vi "Get Torque.vi"(8 "error in (no error)":errorcluster, 11 "HSU MCU V2 in":refnum<class "HSU MCU V2.lvclass">) -> (0 "error out":errorcluster, 2 "Torque":dbl, 3 "HSU MCU V2 out":refnum<class "HSU MCU V2.lvclass">)   [LabVIEW 2024, in "HSU MCU V2.lvclass"]
uses:
  HSU MCU V2.lvclass
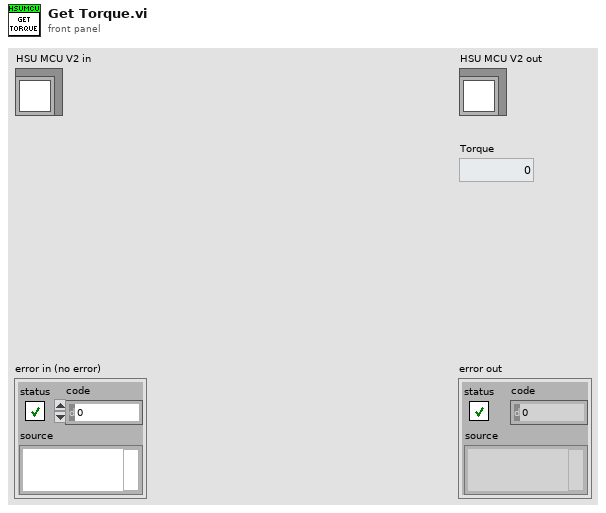
[diagram p1: front panel]
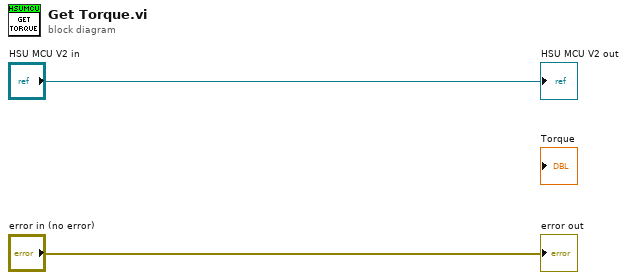
[diagram p0: block diagram]
diagram:
  "error out" <- "error in (no error)"
  "HSU MCU V2 out" <- "HSU MCU V2 in"
